vi "init.vi"(8 "error in (no error)":errorcluster, 10 "Variant":variant, 11 "USB-6000 in":refnum<class "USB-6000.lvclass">) -> (0 "error out":errorcluster, 3 "USB-6000 out":refnum<class "USB-6000.lvclass">)   [LabVIEW 2025, in "USB IO.lvlib" / "USB-6000.lvclass"]
uses:
  USB-6000.lvclass
  USB-6000.lvclass/USB-6000.ctl
  <vilib>/DAQmx/create/channels.llb/DAQmx Create Channel (AI-Voltage-Basic).vi
  <vilib>/DAQmx/create/channels.llb/DAQmx Create Channel (DO-Digital Output).vi
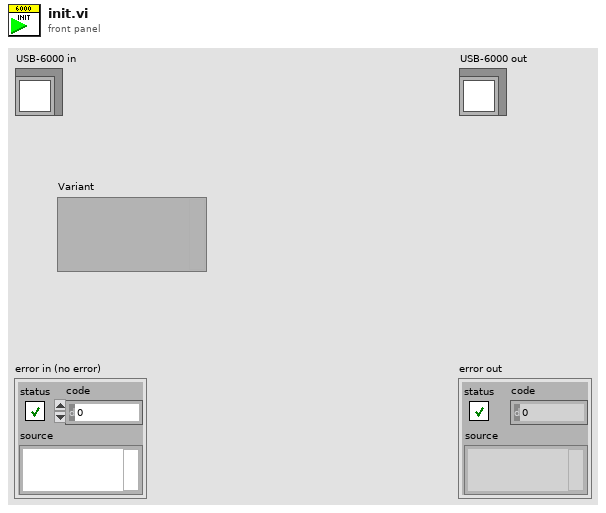
[diagram p1: front panel]
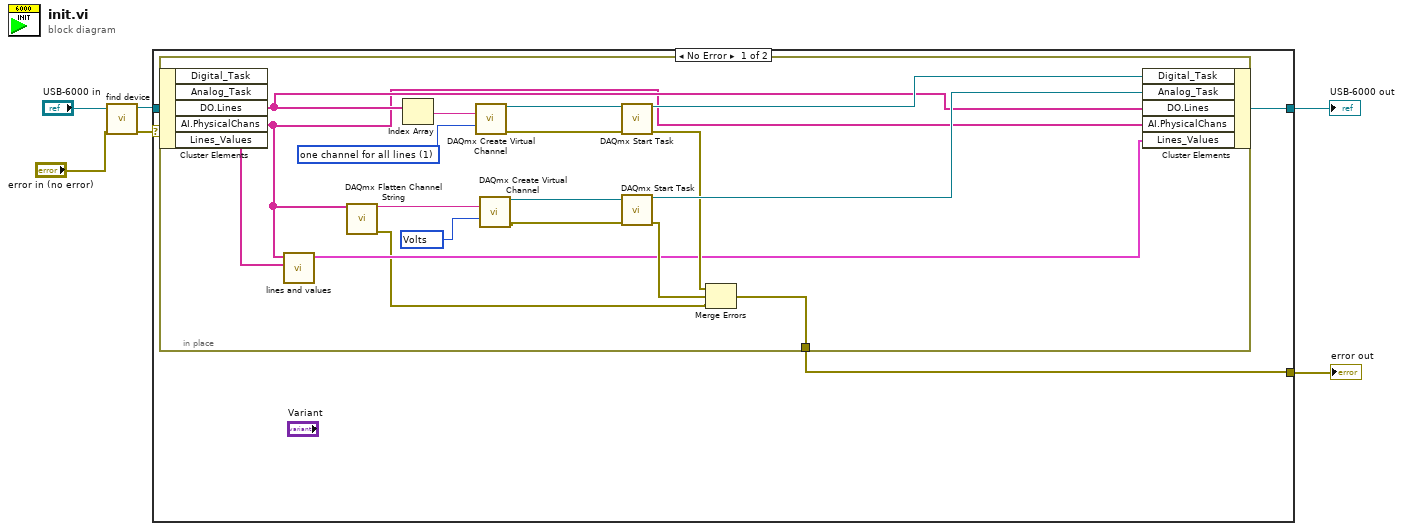
[diagram p0: block diagram]
diagram:
  n1 = call-dynamic "find device.vi"("error in (no error)"="error in (no error)", "USB-6000 in"="USB-6000 in") -> ("error out"=w2:errorcluster, "USB-6000 out"=w3:refnum<class "USB-6000.lvclass">)  [unwired: 8 in]
  n2 = case shown="No Error" w2 {
    selector: w2 -> [_ w28]
    tunnel: [w8 w28] -> w5
    tunnel: [w9 w27] -> w6
    tunnel: w3 -> [w7 w27]
    frame No Error {
      n3 = in-place {
        in-place-border: [w16] -> w8
        w13 = 10348 items=["Volts"=10348, "From Custom Scale"=10065] ("units")
        w26 = 1 items=["one channel for each line", "one channel for all lines"] ("line grouping")
        n4 = in-place-cluster #1(w7) -> ("DO.Lines"=w15:tag[], "AI.PhysicalChans"=w12:tag[])  [unwired: 3 out]
        n5 = call "lines and values.vi"("DO.Lines"=w15, "AI.PhysicalChans"=w12) -> ("Array"=w14:cluster{"Line":string, "Value":i32}[])  [unwired: 9 in]
        n6 = call <vilib>:"DAQmx Flatten Channel String.vi"("names in"=w12) -> ("names out"=w11:string, "error out"=w10:errorcluster)  [unwired: 13 in]
        n7 = Index Array(array=w15) -> (element=w23:tag)  [unwired: 1 in]
        n8 = call-poly <vilib>:"DAQmx Create Virtual Channel.vi"("lines"=w23, "line grouping"=w26) -> ("task out"=w25:refnum<k21>, "error out"=w24:errorcluster)  [unwired: 12 in]
        n9 = call-poly <vilib>:"DAQmx Create Virtual Channel.vi"("physical channels"=w11, "units"=w13) -> ("task out"=w22:refnum<k21>, "error out"=w21:errorcluster)  [unwired: 12 in]
        n10 = call <vilib>:"DAQmx Start Task.vi"("task/channels in"=w25, "error in"=w24) -> ("task out"=w19:refnum<k21>, "error out"=w17:errorcluster)  [unwired: 12 in]
        n11 = call <vilib>:"DAQmx Start Task.vi"("task/channels in"=w22, "error in"=w21) -> ("task out"=w20:refnum<k21>, "error out"=w18:errorcluster)  [unwired: 12 in]
        n12 = Merge Errors(w17, w18, w10) -> (w16:errorcluster)
        n13 = in-place-cluster #1("Digital_Task"=w19, "Analog_Task"=w20, "DO.Lines"=w15, "AI.PhysicalChans"=w12, "Lines_Values"=w14) -> (w9:refnum<class "USB-6000.lvclass">)
      }
    }
    frame Error {
    }
  }
  "error out" <- w5
  "USB-6000 out" <- w6
